vi "hwErrorToSALError.vi"(8 "error in (no error)":errorcluster, 10 "Error Code":i32[](array[numeric]), 11 "Electrometer in":refnum<class "Electrometer.lvclass">) -> (0 "error out":errorcluster, 2 "ErrorArray":T1[](array[typedef]), 3 "Electrometer out":refnum<class "Electrometer.lvclass">)   [LabVIEW 2016, in "Electrometer.lvclass"]
uses:
  Electrometer.lvclass
  ElectrometerError/Controls/errorType.ctl
  ElectrometerError/ElectrometerError.lvclass
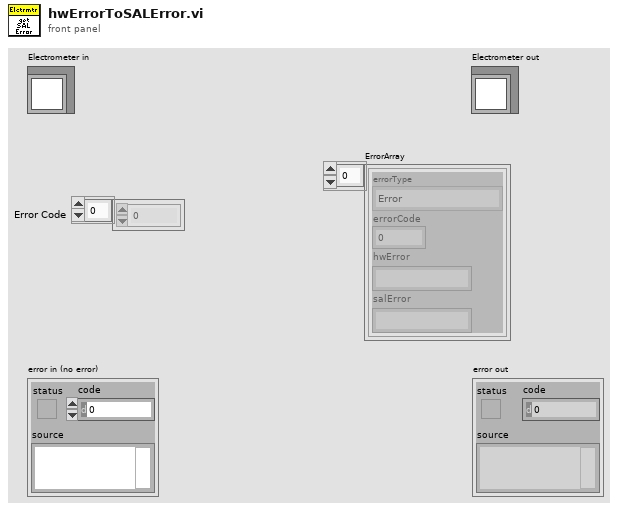
[diagram p1: front panel]
types:
  T1 = typedef "ElectrometerError.lvclass/errorType.ctl" = cluster{"errorType":enum16{"Error", "Warning", "None"}, "errorCode":dbl, "hwError":string, "salError":string}
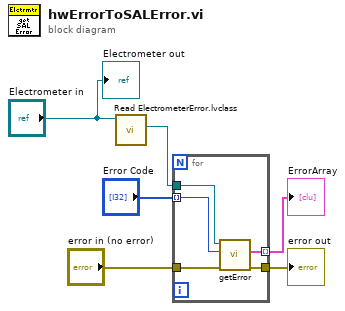
[diagram p0: block diagram]
diagram:
  n1 = call-dynamic "Read ElectrometerError.lvclass.vi"("Electrometer in"="Electrometer in") -> ("ElectrometerError.lvclass"=w4:refnum<class "ElectrometerError.lvclass">)  [unwired: 8 in, 2 out]
  n2 = for {
    tunnel: "Error Code" -> [w10] mode=indexing
    tunnel: w4 -> [w11]
    tunnel: "error in (no error)" -> [w9]
    tunnel: [w8] -> w2
    tunnel: [w7] -> w1 mode=indexing
    n3 = call-dynamic "getError.vi"("error in (no error)"=w9, "errorCode"=w10, "ElectrometerError in"=w11) -> ("error out"=w8:errorcluster, "Error"=w7:T1)  [unwired: 6 in, 1 out]
  }
  "error out" <- w2
  "ErrorArray" <- w1
  "Electrometer out" <- "Electrometer in"
